vi "To Camel Case__ogtk.vi"   [LabVIEW 2016]
doc: "Converts alphabetic characters in string to proper case (i.e., first alphabetic character to uppercase, all others to lowercase for each \"word,\" removing spaces between words)."
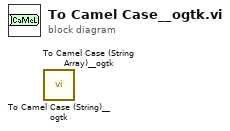
[diagram p0: block diagram]
diagram:
  n1 = call <userlib>:"To Camel Case (String)__ogtk.vi"() -> ()  [unwired: 2 in, 1 out]
  n2 = call <userlib>:"To Camel Case (String Array)__ogtk.vi"() -> ()  [unwired: 2 in, 1 out]
